vi "stream get api information.vi"(8 "error in":errorcluster, 11 "CD in":T1 format="%.0x") -> (0 "error out":errorcluster, 1 "asset ID":string, 2 "dataset name":string, 3 "ID selection":T2, 4 "nominal base url":string, 5 "dataset ID":string, 6 "Channel buffer size":u32=512 min=10 max=1000000, 7 "API key":string)   [LabVIEW 2026, in "Nominal Core Streaming Shared.lvlib"]
uses:
  Nominal Core Streaming Shared.lvlib
  stream configuration mode.ctl
  <vilib>/NI VeriStand/Custom Device API/Custom Device Item Ref.ctl
  Constants.vi
  <vilib>/NI VeriStand/Custom Device API/Custom Device API.lvlib
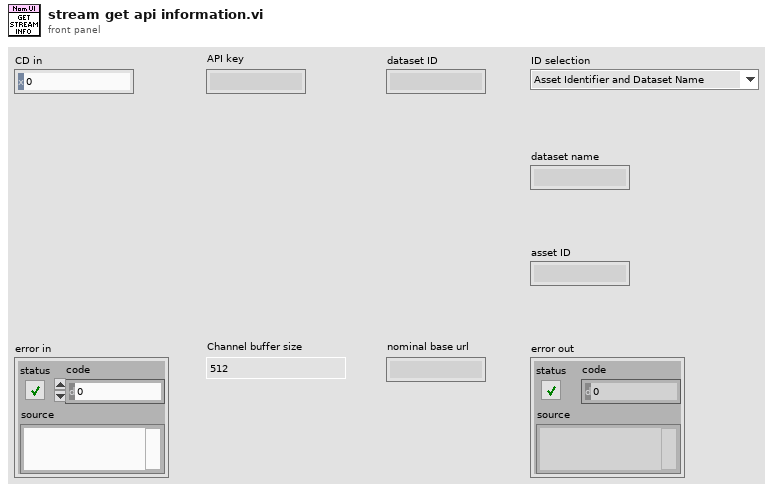
[diagram p1: front panel]
types:
  T1 = typedef "Custom Device API.lvlib/Custom Device Item Ref.ctl" = u64
  T2 = typedef "Nominal Core Streaming Shared.lvlib/stream configuration mode.ctl" = enum16{"Asset Identifier and Dataset Name", "Dataset Identifier"}
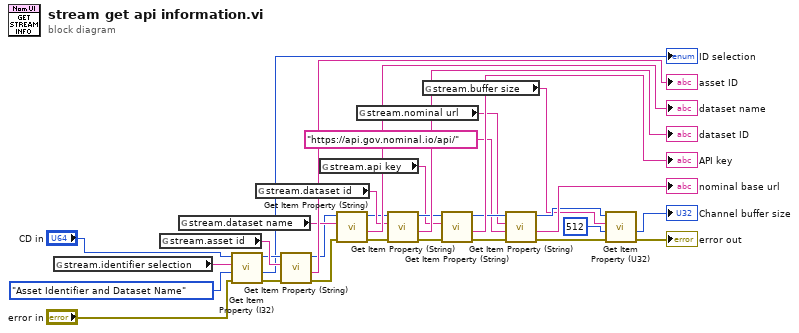
[diagram p0: block diagram]
diagram:
  n1 = global read "Constants.vi" "stream.identifier selection"() -> (w19:string)
  n2 = global read "Constants.vi" "stream.asset id"() -> (w28:string)
  n3 = global read "Constants.vi" "stream.dataset name"() -> (w27:string)
  n4 = call <vilib>:"Get Item Property (I32).vi"("error in (no error)"="error in", "Default Value"=stream_configuration_mode."Asset Identifier and Dataset Name" ("ID selection 2"), "Property Name"=w19, "Item Ref in"="CD in") -> ("error out"=w32:errorcluster, "Value"=→"ID selection":i32, "Item Ref out"=w24:T1)  [unwired: 4 in, 1 out]
  n5 = global read "Constants.vi" "stream.dataset id"() -> (w26:string)
  n6 = call <vilib>:"Get Item Property (String).vi"("error in (no error)"=w32, "Property Name"=w28, "Item Ref in"=w24) -> ("error out"=w23:errorcluster, "Value"=→"asset ID":string, "Item Ref out"=w25:T1)  [unwired: 5 in, 1 out]
  n7 = global read "Constants.vi" "stream.api key"() -> (w14:string)
  n8 = call <vilib>:"Get Item Property (String).vi"("error in (no error)"=w23, "Property Name"=w27, "Item Ref in"=w25) -> ("error out"=w21:errorcluster, "Value"=→"dataset name":string, "Item Ref out"=w22:T1)  [unwired: 5 in, 1 out]
  n9 = global read "Constants.vi" "stream.nominal url"() -> (w8:string)
  n10 = call <vilib>:"Get Item Property (String).vi"("error in (no error)"=w21, "Property Name"=w26, "Item Ref in"=w22) -> ("error out"=w16:errorcluster, "Value"=→"dataset ID":string, "Item Ref out"=w15:T1)  [unwired: 5 in, 1 out]
  n11 = global read "Constants.vi" "stream.buffer size"() -> (w1:string)
  n12 = call <vilib>:"Get Item Property (String).vi"("error in (no error)"=w16, "Property Name"=w14, "Item Ref in"=w15) -> ("error out"=w10:errorcluster, "Value"=→"API key":string, "Item Ref out"=w12:T1)  [unwired: 5 in, 1 out]
  n13 = call <vilib>:"Get Item Property (String).vi"("error in (no error)"=w10, "Default Value"="https://api.gov.nominal.io/api/" ("Nominal Base URL"), "Property Name"=w8, "Item Ref in"=w12) -> ("error out"=w9:errorcluster, "Value"=→"nominal base url":string, "Item Ref out"=w4:T1)  [unwired: 4 in, 1 out]
  n14 = call <vilib>:"Get Item Property (U32).vi"("error in (no error)"=w9, "Default Value"=u32 512, "Property Name"=w1, "Item Ref in"=w4) -> ("error out"=→"error out":errorcluster, "Value"=→"Channel buffer size":u32)  [unwired: 4 in, 2 out]
